vi "Enqueuer Wrapper.vi"() -> (3 "Message Enqueuer out":refnum<class "Message Enqueuer.lvclass">)   [LabVIEW 2016, in "Controller.lvlib" / "gController.lvclass"]
uses:
  gController.lvclass
  <vilib>/ActorFramework/Actor/Actor.lvclass
  <vilib>/ActorFramework/Message Enqueuer/Message Enqueuer.lvclass
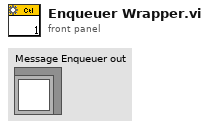
[diagram p1: front panel]
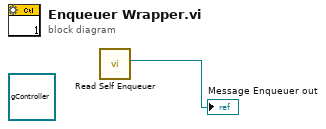
[diagram p0: block diagram]
diagram:
  (unwired) refnum<class "gController.lvclass"> refnum ("Controller.lvlib:gController")
  n1 = call <vilib>:"Read Self Enqueuer.vi"() -> ("Self Enqueuer"=→"Message Enqueuer out":refnum<class "Message Enqueuer.lvclass">)  [unwired: 11 in]
